vi "Convert PL Experiment to ITX Folder.vi"() -> ()   [LabVIEW 2013]
panel:
  in  "wavenames (.Vx, etc)":string[](array[string])=["wavelength", "intensity", "XX", "YY"]
  in  "Notes":string="insert some notes here"
  in  "ITX  path":path=path "P:/users1/Giriraj/20131022_PL_Bo290/PAD 14_2/PL_ITX"
  in  "PL txt Folder Path":path=path "P:/users1/Giriraj/20131022_PL_Bo290/PAD 14_2/PL_txt_PRI"
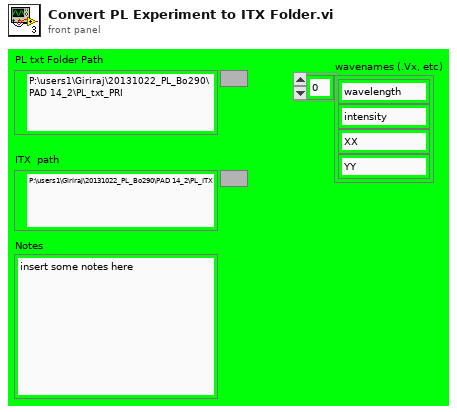
[diagram p1: front panel]
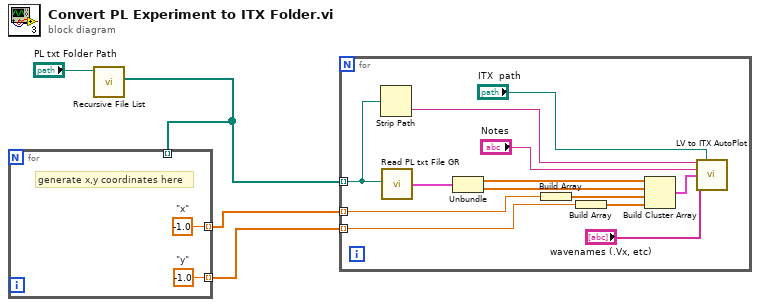
[diagram p0: block diagram]
diagram:
  n1 = call <vilib>:"Recursive File List.vi"("Folder Path"="PL txt Folder Path") -> ("All Files in Dir"=w1:path[])  [unwired: 6 in, 4 out]
  n2 = for {
    tunnel: [w6] -> w3 mode=indexing
    tunnel: [w5] -> w2 mode=indexing
    tunnel: w1 -> [_] mode=indexing
    w5 = -1.0  # "y"
    w6 = -1.0  # "x"
    # "generate x,y coordinates here"
  }
  n3 = for {
    tunnel: w1 -> [w19] mode=indexing
    tunnel: w3 -> [w8] mode=indexing
    tunnel: w2 -> [w7] mode=indexing
    n4 = Strip Path(path=w19) -> (name=w18:string)  [unwired: 1 out]
    n5 = call "Read PL txt File GR.vi"("Path"=w19) -> ("XY Graph"=w16:cluster{"all rows":dbl[], "all rows":dbl[]})
    n6 = Unbundle(w16) -> ("all rows"=w15:dbl[], "all rows"=w14:dbl[])
    n7 = Build Array(w8) -> (w13:dbl[])
    n8 = Build Array(w7) -> (w12:dbl[])
    n9 = Build Cluster Array(w15, w14, w13, w12) -> (w11:cluster{"all rows":dbl[]}[])
    n10 = call <userlib>:"LV to ITX AutoPlot.vi"("filename"=w18, "path"="ITX  path", "Notes"="Notes", "Data"=w11, "wavenames (.Vx, etc)"="wavenames (.Vx, etc)") -> ()  [unwired: 10 in, 1 out]
  }
